vi "WIO Test.vi"() -> ()   [LabVIEW 2019]
uses:
  <userlib>/MicroPython/VIs/uPythonX/uPythonX.xctl
  <userlib>/MicroPython/VIs/SystemLink/Systemlink Tag.xctl
panel:
  in  "Load?":bool=TRUE
  out "Waveform Chart":u32(graph)=1537
  out "Console":string
  in  "stop":bool
  in  "WIO Code":T1(xcontrol)={"VISA Refnum in"="ASRL44::INSTR", "Python Code"="import machine, network, ubinascii, ujson, urequests, utime\nfrom pyb import LED\n\nled = LED(1) # 1=red, 2=green, 3=blue\n\n# Info\n\nKey = \"key\"\n\nurlBase = \"https://api.systemlinkcloud.com/nitag/v2/tags/\"\nGrove = \"https://us.wio.seeed.io/v1/node/GroveTempA0/temp?access_token=7381b4de59f377d0f957db3c9ca13d87\"\n\nurlValue = urlBase + 'fred' + \"/values/current\"\nurlCount = urlBase + 'msec' + \"/values/current\"\n\nheaders = {\"Accept\":\"application/json\",\"x-ni-api-key\":Key}\n     \ndef Update(iteration,LastTick):\n     try:\n          response = urequests.get(Grove)\n          value = response.text\n          response.close()\n     except:\n          print('error')\n     \n     data = ujson.loads(value)\n     Value = data.get(\"temperature\")\n     print (\"value = \",Value)\n     strValue = str(Value)+': ' +str(iteration)\n     propValue = {\"value\":{\"type\":'STRING',\"value\":strValue}}\n\n     try:\n          response = urequests.put(urlValue,headers=headers,json=propValue)\n          print(response.text)\n          response.close()\n     except:\n          print('error')\n\n     time = utime.ticks_ms() - LastTick\n     propValue = {\"value\":{\"type\":'INT',\"value\":str(time)}}\n\n     try:\n          response = urequests.put(urlCount,headers=headers,json=propValue)\n          print(response.text)\n          response.close()\n     except:\n          print('error')\n     led.toggle()\n\ni = 0\nwhile True:\n     old = utime.ticks_ms()\n     print(i)\n     Update(i,old)\n     i = i + 1\n     \n\n\n\n\n\n\n\n\n\n\n\n\n\n\n\n"}
  in  "Systemlink Tag":T2(xcontrol)={"Tag Name"="fred", "Type"="STRING", "Data"="hi"}
  in  "WiFi Code":T1(xcontrol)={"VISA Refnum in"="ASRL44::INSTR", "Python Code"="import machine, network, ubinascii, ujson, urequests, utime\nfrom pyb import LED\n\nWiFi = network.WLAN()\nled = LED(1) # 1=red, 2=green, 3=blue\n\nmac = ubinascii.hexlify(network.WLAN().config(\"mac\"),\":\").decode()\nprint(\"MAC address: \" + mac)\ndef connect():\n     if not WiFi.isconnected():\n          print (\"Connecting ..\")\n          WiFi.active(True)\n          WiFi.connect(\"username\",\"password\")\n          LED(2).on()\n\n          i=0\n          while i < 25 and not WiFi.isconnected():\n               utime.sleep_ms(200)\n               i=i+1\n          if WiFi.isconnected():\n               print (\"Connection succeeded\")\n          else:\n               print (\"Connection failed\")\n\nwhile True:\n     connect()\n     print (\"WiFi: \",WiFi.isconnected())\n     if WiFi.isconnected():\n          LED(2).off()\n          break\n     else:\n          LED(2).on()\n\n\n\n\n\n\n"}
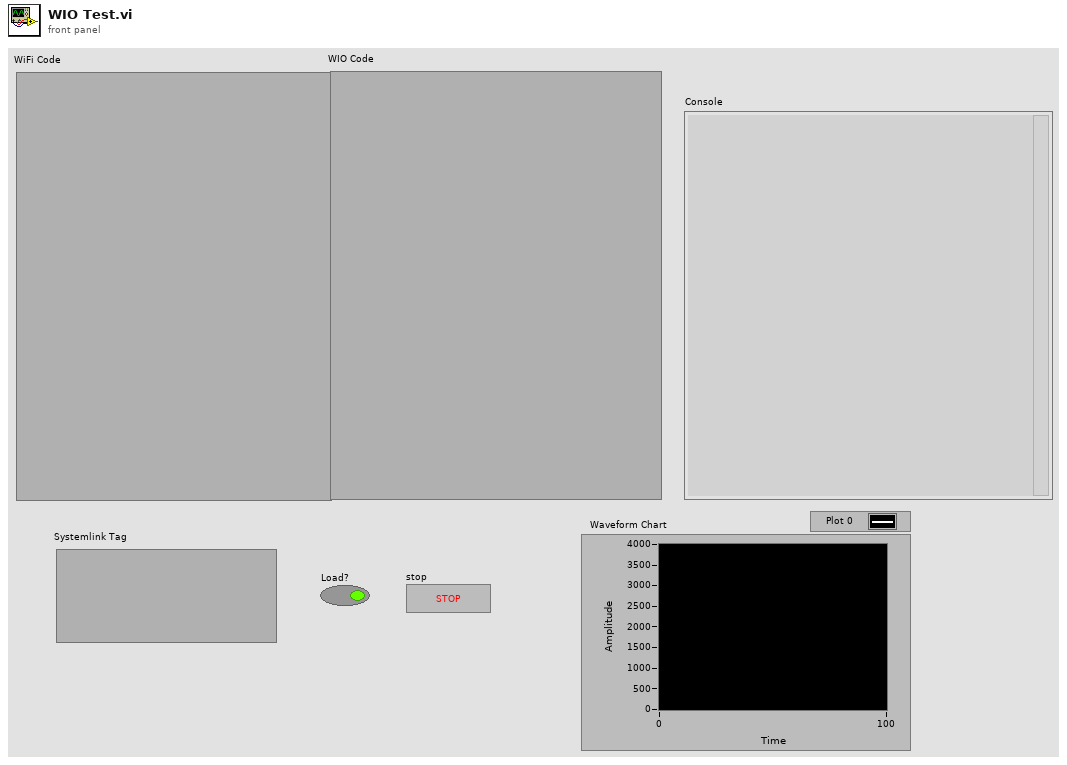
[diagram p1: front panel]
types:
  T1 = cluster{"VISA Refnum in":refnum<visa-resource-name>, "Python Code":string}
  T2 = cluster{"Tag Name":string, "Type":string, "Data":string}
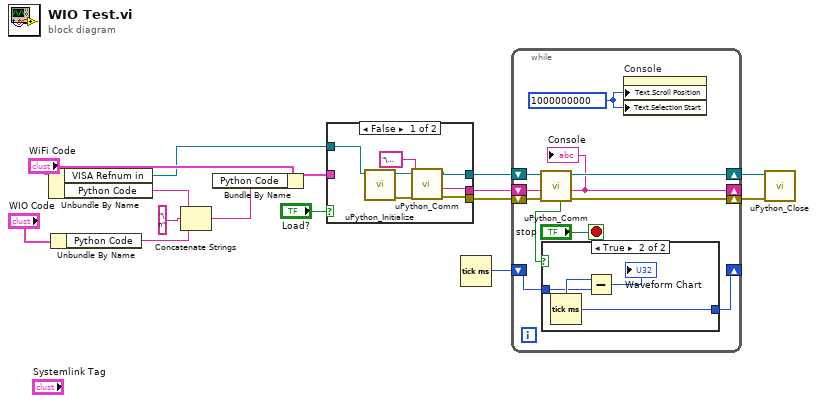
[diagram p0: block diagram]
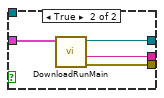
[diagram p2: hidden frame]
diagram:
  n1 = Unbundle By Name("WiFi Code") -> ("VISA Refnum in"=w2:refnum<visa-resource-name>, "Python Code"=w14:string)
  n2 = Unbundle By Name("WIO Code") -> ("Python Code"=w13:string)
  n3 = Concatenate Strings(w14, "\n" ("string"), w13) -> (w10:string)
  n4 = Bundle By Name(cluster="WiFi Code", "Python Code"=w10) -> (w9:T1)
  n5 = case shown="False" "Load?" {
    tunnel: w9 -> [_ w26]
    tunnel: [w18 w25] -> w8
    tunnel: [w20 w24] -> w7
    tunnel: [w17 w23] -> w4
    tunnel: w2 -> [w19 _]
    frame False {
      n6 = call <userlib>:"uPython_Initialize.vi"("VISA Refnum in"=w19) -> ("error out"=w21:errorcluster, "VISA Refnum out"=w22:refnum<visa-resource-name>)  [unwired: 8 in, 1 out]
      n7 = call <userlib>:"uPython_Comm.vi"("error in (no error)"=w21, "Script"="\u0004", "VISA Refnum in"=w22) -> ("error out"=w18:errorcluster, "Console Out"=w17:string, "VISA out"=w20:refnum<visa-resource-name>)  [unwired: 4 in, 2 out]
    }
    frame True {
      n8 = call <userlib>:"DownloadRunMain.vi"("Data In"=w26) -> ("error out"=w25:errorcluster, "Reply"=w23:string, "VISA Refnum out"=w24:refnum<visa-resource-name>)  [unwired: 8 in]
    }
  }
  n9 = Tick Count (ms)() -> (millisecond timer value=w3:u32)
  n10 = while {
    shift-right: [w35] -> w6
    shift-left: w8 -> [w37]
    shift-right: [w34] -> w5
    shift-left: w7 -> [w36]
    shift-right: [w31] -> _
    shift-left: w4 -> [w33]
    shift-right: [w29] -> _
    shift-left: w3 -> [w28]
    stop <- "stop" stop-if-true
    w30 = u32 1000000000 ("Text.Selection:Start")
    n11 = call <userlib>:"uPython_Comm.vi"("error in (no error)"=w37, "Console In"=w33, "VISA Refnum in"=w36) -> ("error out"=w35:errorcluster, "Console Out"=w31:string, "VISA out"=w34:refnum<visa-resource-name>, "Update?"=w27:bool)  [unwired: 4 in, 1 out]
    "Console" <- w31
    n12 = case shown="True" w27 {
      tunnel: [w38 w41] -> w29
      tunnel: w28 -> [w38 w40]
      frame False {
      }
      frame True {
        n13 = Tick Count (ms)() -> (millisecond timer value=w41:u32)
        n14 = Subtract(x=w41, y=w40) -> (x-y=→"Waveform Chart":u32)
      }
    }
    n15 = property on="Console" class="Str"("Text.Scroll Position"=w30, "Text.Selection Start"=w30) -> ()  [unwired: 2 in, 2 out]
  }
  n16 = call <userlib>:"uPython_Close.vi"("error in"=w6, "VISA  in"=w5) -> ()  [unwired: 8 in, 2 out]
